vi "EQE_CloseShutter.vi"() -> (0 "Error Code":i32)   [LabVIEW 2017]
uses:
  Program Files (x86)/Bentham/SDK/code examples/LabView/8.0/BenHw/benhw32_stdcall.dll
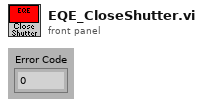
[diagram p1: front panel]
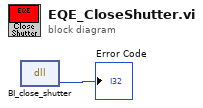
[diagram p0: block diagram]
diagram:
  n1 = dll-call lib="C:/Program Files (x86)/Bentham/SDK/code examples/LabView/8.0/BenHw/benhw32_stdcall.dll" fn="BI_close_shutter"() -> ("return type"=→"Error Code":i32)  [unwired: 3 in, 2 out]
